vi "Verify Firmware.vi"() -> ()   [LabVIEW 2020]
doc: "This Vi will upgrade the RT device's firmware if it is not supported by SystemLink Client, which means firmware must be higher than version 6."
uses:
  Users/josferna/OneDrive - NI/Documents/Accounts&Proojects/Open Case Files/01072359 - Microsoft/rad-master/subVIs/Targets/TypeDefs/rad_Target Network Settings.ctl
  <vilib>/nisyscfg/Firmware Status.ctl
  <vilib>/nisyscfg/Upgrade Firmware (File).vi
  <vilib>/nisyscfg/Close (Hardware).vi
  <vilib>/nisyscfg/Close (System).vi
  <resource>/objmgr/nisysapi.rc
  <vilib>/nisyscfg/nisyscfg.lvlib
panel:
  in  "error in":errorcluster caption="error in (no error)"
  out "error out":errorcluster
  out "Firmware Status":T1=2 items=["update pending auto restart"=-4, "verifying new image"=-3, "writing/flashing new image"=-2, "waiting for image"=-1, "corrupt firmware, cannot run"=0, "no firmware installed"=1, ""=2, "update pending user restart"=3, "update pending user action"=4, "update attempt failed"=5]
  out "Detailed Result":string
  in  "Firmware File":path=path "C:/Program Files (x86)/National Instruments/Shared/Firmware/cRIO/76D6/cRIO-9068_8.5.0.cfg"
  in  "Target information":T3={"Hostname"="", "Serial number"="", "Product name"="", "Product code"=0, "System status"="", "Credential type"=enum."None/Unlocked", "User added?"=FALSE, "Primary NIC"={"MAC address"="", "IP Address Request Mode"=2, "IP address"="", "Subnet mask"="", "Gateway"="", "DNS server"=""}} {"Primary NIC"."IP Address Request Mode" items=["Static"=1, "DHCP/Link-Local"=2, "Link-Local Only"=4, "DHCP Only"=8]}
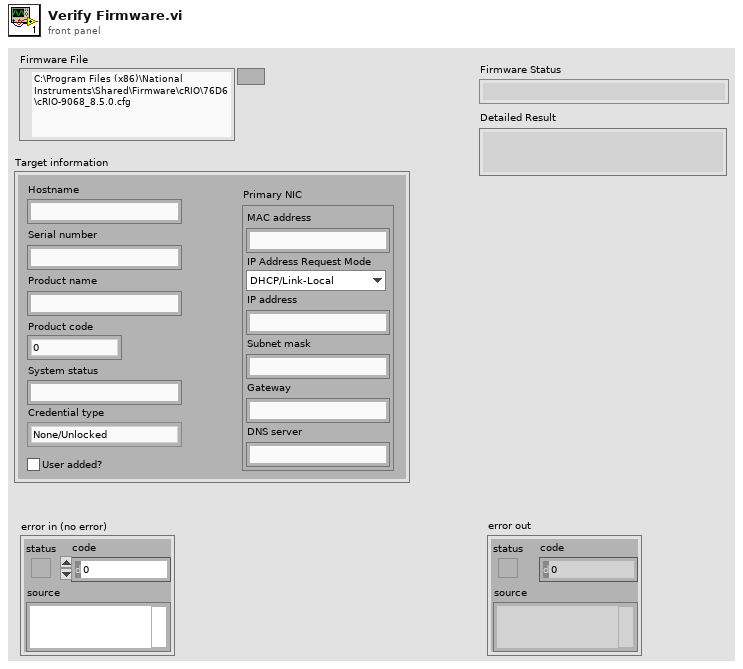
[diagram p1: front panel]
types:
  T1 = typedef "nisyscfg.lvlib/Firmware Status.ctl" = i32
  T2 = typedef "rad_Target Network Settings.ctl" = cluster{"MAC address":string, "IP Address Request Mode":i32, "IP address":string, "Subnet mask":string, "Gateway":string, "DNS server":string}
  T3 = cluster{"Hostname":string, "Serial number":string, "Product name":string, "Product code":i32, "System status":string, "Credential type":enum16{"None/Unlocked", "FTP Password", "NIAuth Credentials"}, "User added?":bool, "Primary NIC":T2}
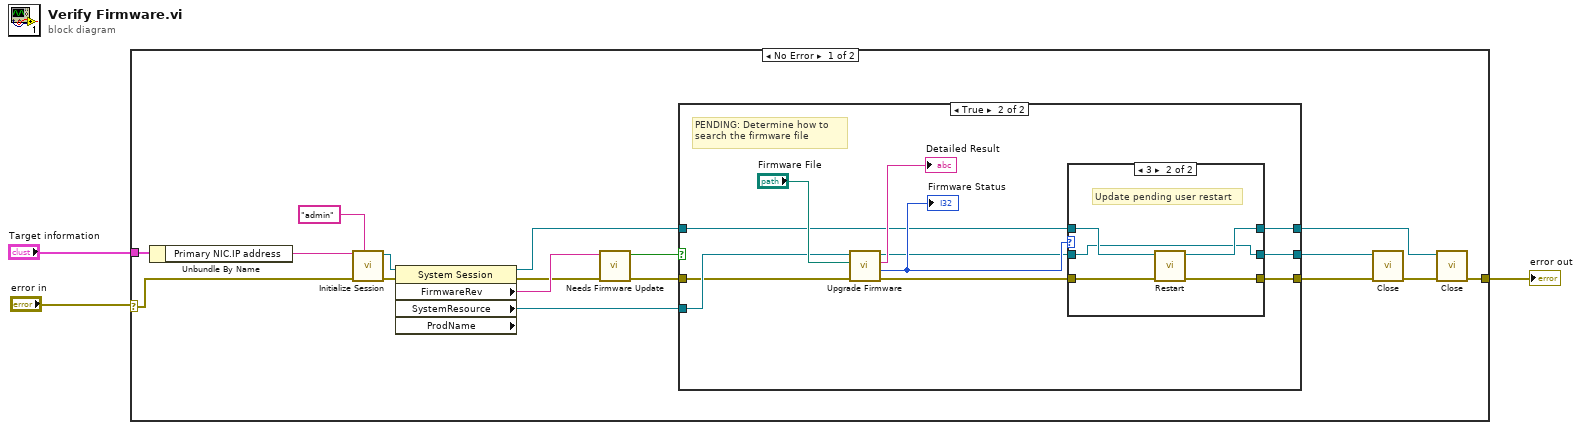
[diagram p0: block diagram]
diagram:
  n1 = case shown="No Error" "error in" {
    selector: "error in" -> [w4 w43]
    tunnel: [w20 w43] -> w3
    tunnel: "Target information" -> [w13 _]
    frame No Error {
      n2 = Unbundle By Name(w13) -> ("Primary NIC.IP address"=w12:string)
      n3 = call <vilib>:"Initialize Session.vi"("User Name"="admin", "error in (no error)"=w4, "Target (localhost)"=w12) -> ("error out"=w16:errorcluster, "Session out"=w15:refnum<k21>)  [unwired: 7 in]
      n4 = property class="System Session" props=["FirmwareRev", "SystemResource", "ProdName"](reference=w15, error in=w16) -> (reference out=w7:refnum<k21>, error out=w10:errorcluster, "FirmwareRev"=w11:string, "SystemResource"=w14:refnum<k20>)  [unwired: 1 out]
      n5 = call "Needs Firmware Update.vi"("error in (no error)"=w10, "FirmwareRev"=w11) -> ("error out"=w8:errorcluster, "Update?"=w9:bool)  [unwired: 8 in]
      n6 = case shown="True" w9 {
        tunnel: [w22 w24] -> w19
        tunnel: [w23 w27] -> w18
        tunnel: w14 -> [w22 w32]
        tunnel: w8 -> [w23 w31]
        tunnel: w7 -> [w21 w28]
        tunnel: [w21 w26] -> w5
        frame False {
        }
        frame True {
          # "PENDING: Determine how to\nsearch the firmware file"
          n7 = call-poly <vilib>:"Upgrade Firmware.vi"("error in (no error)"=w31, "Firmware File"="Firmware File", "Resource in"=w32) -> ("error out"=w30:errorcluster, "Firmware Status"=w29:T1, "Detailed Result"=→"Detailed Result":string, "Resource out"=w25:refnum<k20>)  [unwired: 5 in]
          "Firmware Status" <- w29
          n8 = case shown="3" w29 {
            tunnel: w30 -> [w36 w42]
            tunnel: w28 -> [w37 w41]
            tunnel: [w37 w40] -> w26
            tunnel: [w36 w39] -> w27
            tunnel: w25 -> [w35 w38]
            tunnel: [w35 w38] -> w24
            frame 0, Default {
            }
            frame 3 {
              # "Update pending user restart"
              n9 = call <vilib>:"Restart.vi"("error in (no error)"=w42, "Session in"=w41) -> ("error out"=w39:errorcluster, "Session out"=w40:refnum<k21>)  [unwired: 7 in, 1 out]
            }
          }
        }
      }
      n10 = call-poly <vilib>:"Close.vi"("error in (no error)"=w18, "Resource in"=w19) -> ("error out"=w6:errorcluster)  [unwired: 9 in]
      n11 = call-poly <vilib>:"Close.vi"("error in (no error)"=w6, "Session in"=w5) -> ("error out"=w20:errorcluster)  [unwired: 9 in]
    }
    frame Error {
    }
  }
  "error out" <- w3
